vi "Get settings.vi"(0 "MODULE ADDRESS":i32=1, 2 "PORT NAME":string="Inlet_Heaters") -> (8 "Settings":string[](array[string]), 9 "Error":bool, 10 "Comments":string)   [LabVIEW 2010]
panel:
  out "Delimiters found":i32[](array[numeric])
  in  "No of Locations":i32[](array[numeric])=[380, 241]
  out "String":string
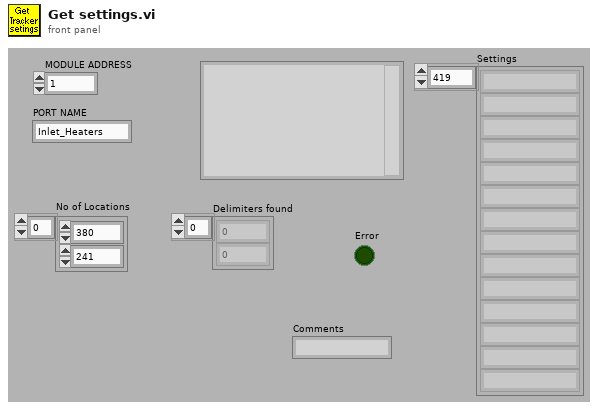
[diagram p1: front panel]
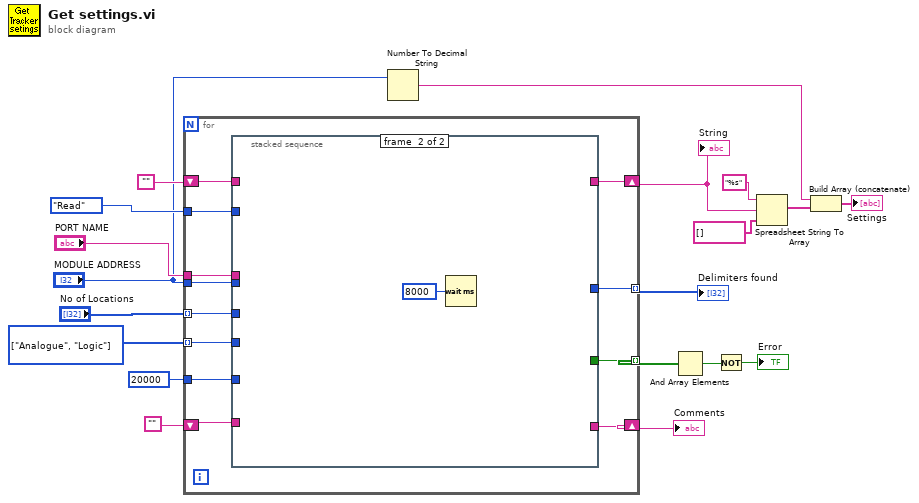
[diagram p0: block diagram]
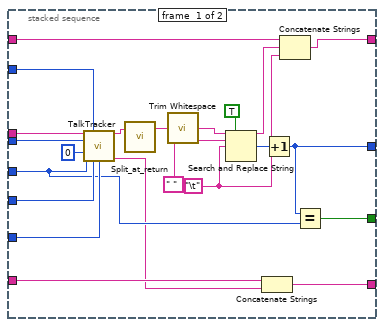
[diagram p2: hidden frame]
diagram:
  w16 = enum16{"Logic", "Analogue"}[] [enum."Analogue", enum."Logic"] items=["Logic", "Analogue"]
  n1 = for {
    tunnel: "MODULE ADDRESS" -> [w31]
    tunnel: "PORT NAME" -> [w30]
    tunnel: enum16{"Set", "Read"}."Read" ("Set") -> [w29]
    tunnel: u32 20000 ("Timeout/ms") -> [w28]
    tunnel: [w20] -> w14 mode=indexing
    tunnel: w16 -> [w27] mode=indexing
    tunnel: "No of Locations" -> [w24] mode=indexing
    shift-right: [w26] -> w12
    shift-left: "" -> [w25]
    tunnel: [w23] -> w5 mode=indexing
    shift-right: [w22] -> w1
    shift-left: "" -> [w21]
    n2 = stacked-sequence {
      tunnel: w31 -> [w53 _]
      tunnel: w30 -> [w52 _]
      tunnel: w29 -> [w51 _]
      tunnel: w28 -> [w49 _]
      tunnel: w27 -> [w46 _]
      tunnel: [w44 _] -> w26
      tunnel: w25 -> [w43 _]
      tunnel: w24 -> [w40 _]
      tunnel: [w39 _] -> w23
      tunnel: [w38 _] -> w22
      tunnel: w21 -> [w37 _]
      tunnel: [w32 _] -> w20
      frame #0 {
        w42 = "\t"
        n3 = call "TalkTracker.vi"("PORT NAME"=w52, "Set"=w51, "MODULE ADDRESS"=w53, "LOCATION"=0, "NO. LOCATIONS"=w40, "Analogue"=w46, "Timeout/ms"=w49) -> ("Response"=w35:string, "Comment out"=w36:string)  [unwired: 6 in, 1 out]
        n4 = call "Split_at_return.vi"("String"=w35) -> ("before substring"=w34:string)  [unwired: 1 in, 3 out]
        n5 = call <vilib>:"Trim Whitespace.vi"("string"=w34) -> ("trimmed string"=w33:string)  [unwired: 1 in]
        n6 = Search and Replace String(replace all?=TRUE ("replace all? (F)"), input string=w33, search string=" ", replace string=w42) -> (result string=w45:string, number of replacements=w41:i32)  [unwired: 4 in, 2 out]
        n7 = Concatenate Strings(w37, w36) -> (w38:string)
        n8 = Increment(x=w41) -> (x+1=w32:i32)
        n9 = Concatenate Strings(w43, w45, w42) -> (w44:string)
        n10 = Equal?(x=w32, y=w40) -> (x = y?=w39:bool)
      }
      frame #1 {
        n11 = Wait (ms)(milliseconds to wait=u32 8000) -> ()  [unwired: 1 out]
      }
    }
  }
  "String" <- w12
  "Delimiters found" <- w14
  "Comments" <- w1
  n12 = Number To Decimal String(number="MODULE ADDRESS") -> (decimal integer string=w8:string)  [unwired: 1 in]
  n13 = And Array Elements(Boolean array=w5) -> (logical AND=w4:bool)
  n14 = Not(x=w4) -> (.not. x?=→"Error":bool)
  n15 = Spreadsheet String To Array(format string="%s", spreadsheet string=w12, array type (2D Dbl)=string[] []) -> (array=w10:string[])  [unwired: 1 in]
  n16 = Build Array (concatenate)(w8, w10) -> (→"Settings":string[])
